vi "startMotor.vi"(1 "MXP Port":enum16{"A", "B"}(ring), 2 "ID":u32 format="%x") -> (0 "SPI Config Out":T1)   [LabVIEW 2019]
uses:
  SPI/SPI Config.ctl
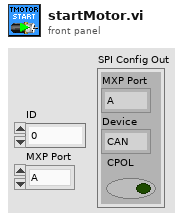
[diagram p1: front panel]
types:
  T1 = typedef "SPI Config.ctl" = cluster{"MXP Port":enum16{"A", "B"}, "Device":enum16{"CAN", "ENC", "IMU1", "IMU2"}, "CPOL":bool}
  T2 = enum16{"100kBPS", "250kBPS", "500kBPS", "1000kBPS"}
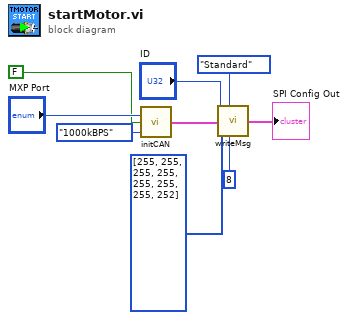
[diagram p0: block diagram]
diagram:
  n1 = call "initCAN.vi"("Baud Rate"=T2."1000kBPS", "CPOL"=FALSE, "MXP Port"="MXP Port") -> ("SPI Config Out"=w4:T1)
  n2 = call "writeMsg.vi"("ID"="ID", "ID Type"=enum16{"Standard", "Extended"}."Standard", "SPI Config In"=w4, "Data to Write"=u8[] [255, 255, 255, 255, 255, 255, 255, 252], "Frames to Write"=u8 8) -> ("SPI Config Out"=→"SPI Config Out":T1)
